vi "Sensirion Flow Meter Read SubVI 08-21-15.vi"(11 "COMPort":u16=20) -> (3 "MeasureResult Scaled":dbl)   [LabVIEW 2015]
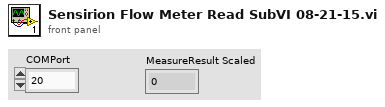
[diagram p1: front panel]
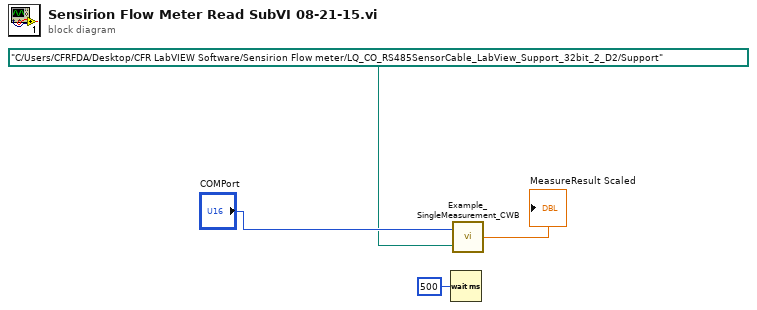
[diagram p0: block diagram]
diagram:
  n1 = Wait (ms)(milliseconds to wait=u32 500) -> ()  [unwired: 1 out]
  n2 = call "Example_SingleMeasurement_CWB.vi"("base path"=path "C:/Users/CFRFDA/Desktop/CFR LabVIEW Software/Sensirion Flow meter/LQ_CO_RS485SensorCable_LabView_Support_32bit_2_D2/Support", "COMPort"="COMPort") -> ("MeasureResult Scaled"=→"MeasureResult Scaled":dbl)
